vi "PCO_SetCmosLineTiming.vi"(7 "dwLineTime":u32, 8 "error in (no error)":errorcluster {"code" format="%x"}, 9 "wTimeBase":u16(ring)=2 items=["ns", "us", "ms"], 10 "wParameter":u16(ring) items=["OFF", "ON"], 11 "ph":u64) -> (0 "error out":errorcluster {"code" format="%x"}, 2 "ErrorMessage":i32 format="%x", 3 "ph out":u64)   [LabVIEW 2020, in "SDK.lvlib" / "SpecialCommandsEdge.lvlib"]
doc: "<b>Description:</b>\nThis function enables or disables the Lightsheet scanning mode of the pco.edge. In Lightsheet scanning mode exposure and delay time setting is correlated to the sensor line time. If this mode is enabled, timing related settings from the functions in TIMING CONTROL can not be used.\nThe setting of delay time and exposure time must be done with the function PCO_SetCmosLineExposureDelay.\nThe resulting exposure-time can be calculated as:\ndwExposureLines*dwLineTime*(1000ˆdwTimebase)\nThe command is only available in operation mode Rolling Shutter.\nThe preferred SCCMOS Readout format is SCCMOS_FORMAT_TOP_BOTTOM\n\n<b>Supported camera type:</b>\npco.edge with Camera Link interface\n\n<b>Descriptor dependency:</b>\nNone"
uses:
  SpecialCommandsEdge.lvlib
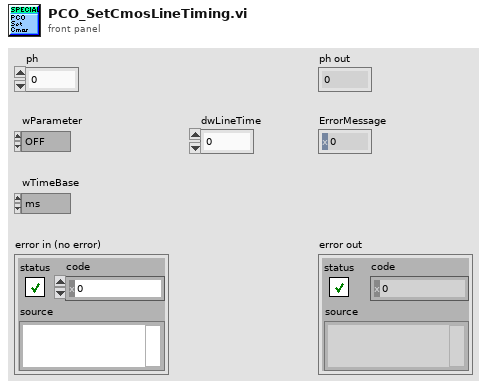
[diagram p1: front panel]
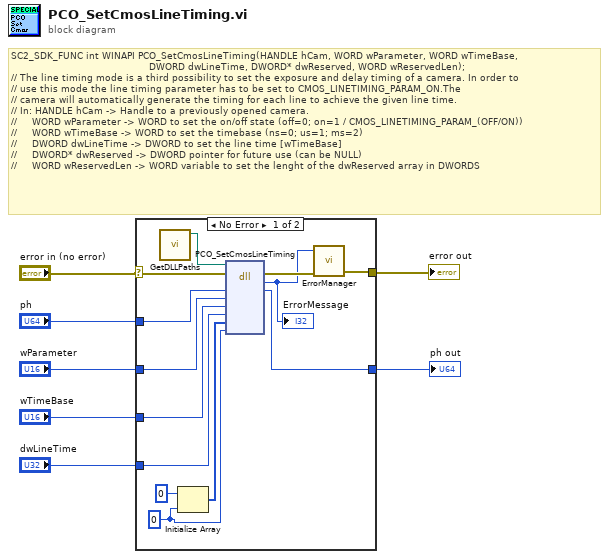
[diagram p0: block diagram]
diagram:
  # "SC2_SDK_FUNC int WINAPI PCO_SetCmosLineTiming(HANDLE hCam, WORD wParameter, WORD wTimeBase,\n                                              DWORD dwLineTime, DWORD* dwReserved, WORD wReservedLen);\n// The line timing mode is a third possibility to set the exposure and delay timing of a camera. In order to \n// use this mode the line timing parameter has to be set to CMOS_LINETIMING_PARAM_ON.The\n// camera will automatically generate the timing for each line to achieve the given line time.\n// In: HANDLE hCam -> Handle to a previously opened camera.\n//     WORD wParameter -> WORD to set the on/off state (off=0; on=1 / CMOS_LINETIMING_PARAM_(OFF/ON))\n//     WORD wTimeBase -> WORD to set the timebase (ns=0; us=1; ms=2)\n//     DWORD dwLineTime -> DWORD to set the line time [wTimeBase]\n//     DWORD* dwReserved -> DWORD pointer for future use (can be NULL)\n//     WORD wReservedLen -> WORD variable to set the lenght of the dwReserved array in DWORDS"
  n1 = case shown="No Error" "error in (no error)" {
    selector: "error in (no error)" -> [w12 w22]
    tunnel: "ph" -> [w20 w21]
    tunnel: [w19 w21] -> w6
    tunnel: "wParameter" -> [w18 _]
    tunnel: "wTimeBase" -> [w17 _]
    tunnel: "dwLineTime" -> [w16 _]
    tunnel: [w10 w22] -> w2
    frame No Error {
      w13 = u16 0 ("dimension size")
      n2 = call "GetDLLPaths.vi"() -> ("SC2_Cam_Path"=w8:path)  [unwired: 9 in, 2 out]
      n3 = Initialize Array(u32 0, w13) -> (w14:u32[])
      n4 = dll-call lib="?" fn="PCO_SetCmosLineTiming"(path in=w8, error in=w12, "ph"=w20, "wParameter"=w18, "wTimeBase"=w17, "dwLineTime"=w16, "dwReserved"=w14, "wReservedLen"=w13) -> (error out=w11:errorcluster, "return type"=w9:i32, "ph"=w19:u64)  [unwired: 6 in, 1 out]
      "ErrorMessage" <- w9
      n5 = call "ErrorManager.vi"("error in (no error)"=w11, "error code"=w9) -> ("error out"=w10:errorcluster)  [unwired: 3 in]
    }
    frame Error {
    }
  }
  "ph out" <- w6
  "error out" <- w2
